vi "FT10_Log LVM Values.vi"(8 "error in (no error)":errorcluster, 10 "Log Cluster in":T1, 11 "Log Loop Cluster in":T5) -> (0 "error out":errorcluster, 1 "Waveform filename":string, 2 "Log Cluster out":T1, 3 "Log Loop Cluster out":T5)   [LabVIEW 2015]
uses:
  Controls/Control_Log Loop Cluster.ctl
  Controls/Control_Log TDMS Filename.ctl
  Controls/Control_Log t0.ctl
  Controls/Control_Log Cluster.ctl
  Controls/Control_Log Time.ctl
  Controls/Control_Log Waveform Cluster.ctl
  Controls/Control_Log Analysis Cluster.ctl
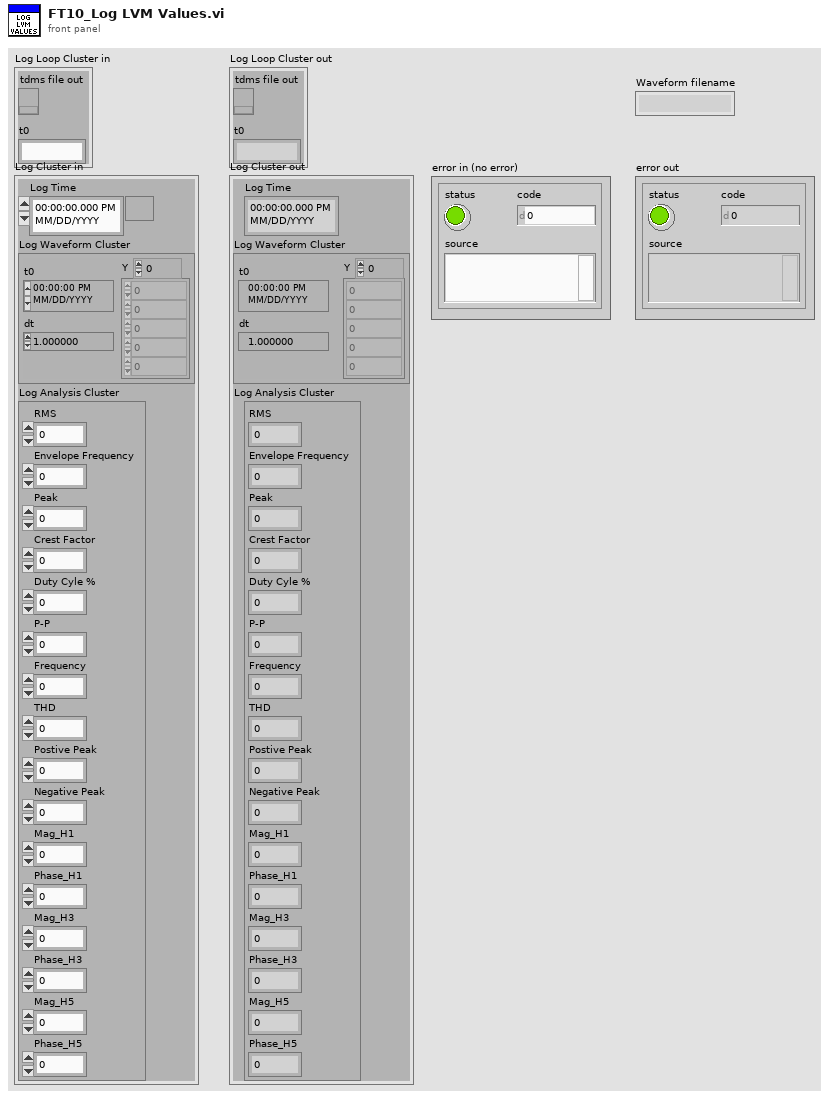
[diagram p1: front panel]
types:
  T1 = typedef "Control_Log Cluster.ctl" = cluster{"Log Time":T2, "Log Waveform Cluster":T3, "Log Analysis Cluster":T4}
  T2 = typedef "Control_Log Time.ctl" = timestamp
  T3 = typedef "Control_Log Waveform Cluster.ctl" = waveform(dbl)
  T4 = typedef "Control_Log Analysis Cluster.ctl" = cluster{"RMS":dbl, "Envelope Frequency":dbl, "Peak":dbl, "Crest Factor":dbl, "Duty Cyle %":dbl, "P-P":dbl, "Frequency":dbl, "THD":dbl, "Postive Peak":dbl, "Negative Peak":dbl, "Mag_H1":dbl, "Phase_H1":dbl, "Mag_H3":dbl, "Phase_H3":dbl, "Mag_H5":dbl, "Phase_H5":dbl}
  T5 = typedef "Control_Log Loop Cluster.ctl" = cluster{"tdms file out":T6, "t0":T7}
  T6 = typedef "Control_Log TDMS Filename.ctl" = refnum<k34>
  T7 = typedef "Control_Log t0.ctl" = string
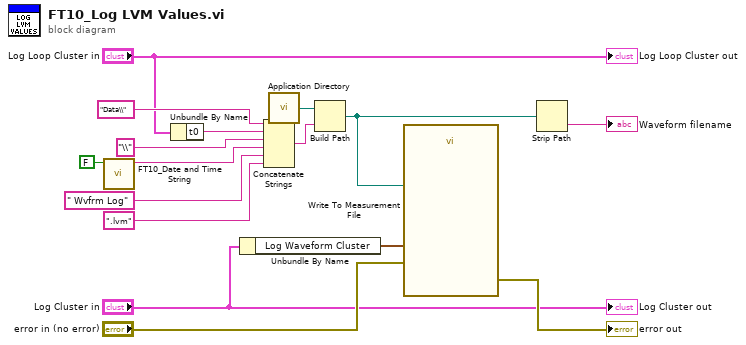
[diagram p0: block diagram]
diagram:
  n1 = call "FT10_Date and Time String.vi"("to UTC"=FALSE) -> ("Date & Time string"=w10:string)  [unwired: 10 in]
  n2 = Unbundle By Name("Log Loop Cluster in") -> ("t0"=w1:T7)
  n3 = Unbundle By Name("Log Cluster in") -> ("Log Waveform Cluster"=w6:T3)
  n4 = Concatenate Strings("Data\\" ("string"), w1, "\\" ("string"), w10, " Wvfrm Log" ("name or relative path"), ".lvm" ("string")) -> (w15:string)
  n5 = call <vilib>:"Application Directory.vi"() -> ("Application Directory"=w16:path)
  n6 = Build Path(base path=w16, name or relative path=w15) -> (appended path=w4:path)
  n7 = call "Write To Measurement File"("Signals"=w6, "error in (no error)"="error in (no error)", "Filename"=w4) -> ("error out"=→"error out":errorcluster)  [unwired: 14 in, 2 out]
  n8 = Strip Path(path=w4) -> (name=→"Waveform filename":string)  [unwired: 1 out]
  "Log Loop Cluster out" <- "Log Loop Cluster in"
  "Log Cluster out" <- "Log Cluster in"
